vi "IncrementarCuenta_&checkFinal.vi"(8 "error in (no error)":errorcluster, 11 "TEST ASICS INPUT in":T1={"COORD. IN X"=0, "COORD IN Y"=0, "COORD OK X"=0, "COORD OK Y"=0, "COORD NOK X"=0, "COORD NOK Y"=0, "NºASICS A TESTEAR"=0, "SELECCIÓN DE TEST"=enum."TEST ASICS LST", "CUENTA ASICS"=0, "OPERADOR"="Javier Morales"}) -> (0 "error out":errorcluster, 1 "Asics pendientes":u32, 2 "FINAL ASICS??":bool, 3 "TEST ASICS INPUT out":T1={"COORD. IN X"=0, "COORD IN Y"=0, "COORD OK X"=0, "COORD OK Y"=0, "COORD NOK X"=0, "COORD NOK Y"=0, "NºASICS A TESTEAR"=0, "SELECCIÓN DE TEST"=enum."TEST ASICS LST", "CUENTA ASICS"=0, "OPERADOR"="Javier Morales"})   [LabVIEW 2019]
uses:
  Type_defs/INPUT TEST.ctl
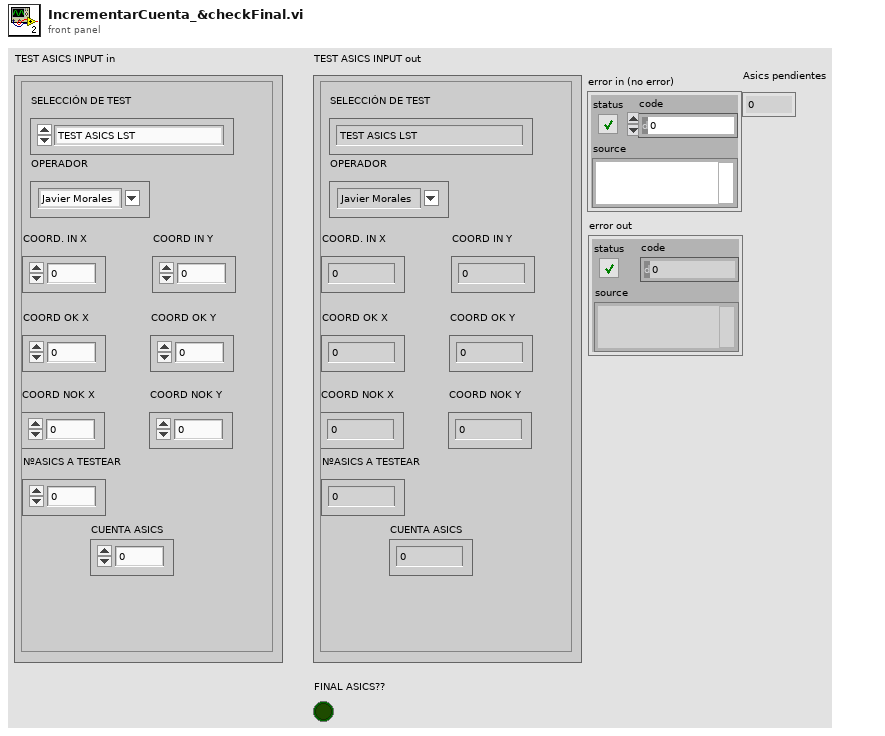
[diagram p1: front panel]
types:
  T1 = typedef "INPUT TEST.ctl" = cluster{"COORD. IN X":u16, "COORD IN Y":u16, "COORD OK X":u16, "COORD OK Y":u16, "COORD NOK X":u16, "COORD NOK Y":u16, "NºASICS A TESTEAR":u32, "SELECCIÓN DE TEST":enum16{"TEST ASICS LST"}, "CUENTA ASICS":u32, "OPERADOR":string}
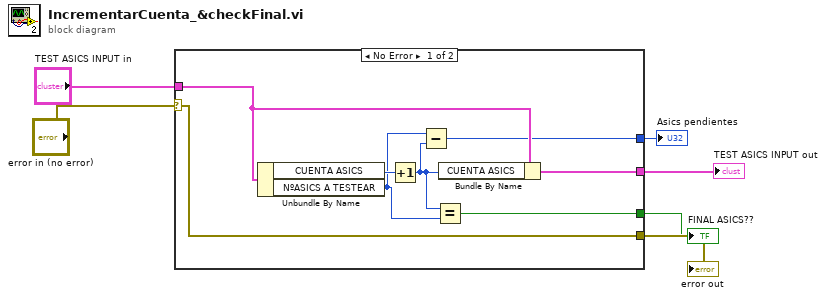
[diagram p0: block diagram]
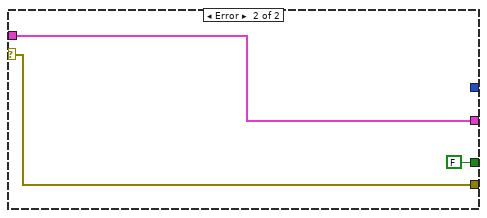
[diagram p2: hidden frame]
diagram:
  n1 = case shown="No Error" "error in (no error)" {
    selector: "error in (no error)" -> [w11 w17]
    tunnel: [w14 w16] -> w6
    tunnel: "TEST ASICS INPUT in" -> [w13 w16]
    tunnel: [w11 w17] -> w3
    tunnel: [w10 FALSE] -> w2
    tunnel: [w7 _] -> w1
    frame No Error {
      n2 = Unbundle By Name(w13) -> ("CUENTA ASICS"=w12:u32, "NºASICS A TESTEAR"=w9:u32)
      n3 = Increment(x=w12) -> (x+1=w8:u32)
      n4 = Subtract(x=w9, y=w8) -> (x-y=w7:u32)
      n5 = Equal?(x=w8, y=w9) -> (x = y?=w10:bool)
      n6 = Bundle By Name(cluster=w13, "CUENTA ASICS"=w8) -> (w14:T1)
    }
    frame Error {
    }
  }
  "TEST ASICS INPUT out" <- w6
  "error out" <- w3
  "FINAL ASICS??" <- w2
  "Asics pendientes" <- w1
